vi "Send Stop Event.vi"(8 "error in (no error)":errorcluster, 11 "View In":refnum<class "View.lvclass">) -> (0 "error out":errorcluster, 3 "View Out":refnum<class "View.lvclass">)   [LabVIEW 2020, in "View.lvclass"]
uses:
  View.lvclass
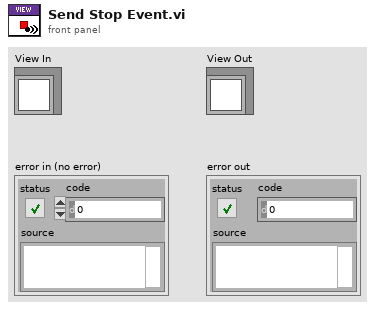
[diagram p1: front panel]
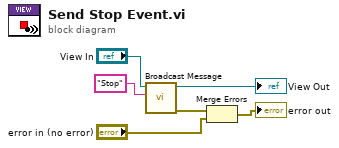
[diagram p0: block diagram]
diagram:
  n1 = call-dynamic "Broadcast Message.vi"("Message"="Stop", "Process In"="View In") -> ("error out"=w3:errorcluster, "Process Out"=→"View Out":refnum<class "View.lvclass">)  [unwired: 8 in]
  n2 = Merge Errors(w3, "error in (no error)") -> (→"error out":errorcluster)
